vi "Example ADC PCF8591.vi"() -> ()   [LabVIEW 2014]
uses:
  vi.lib/Q-WaveSystems/QwaveSys Raspberry Pi for LabVIEW Home-Education/QwaveSys Raspberry Pi Library.lvlib
panel:
  in  "DAC":u8=77
  out "A3":i32
  out "A2":i32
  out "A1":i32
  out "A0":i32
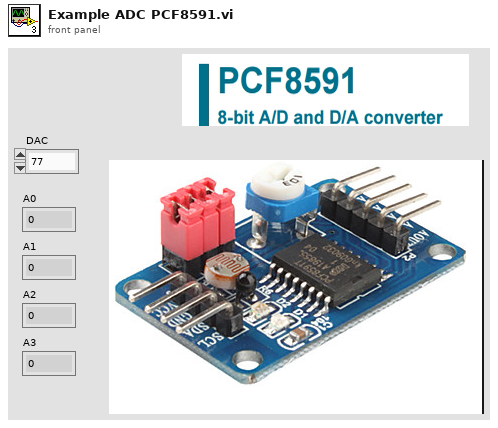
[diagram p1: front panel]
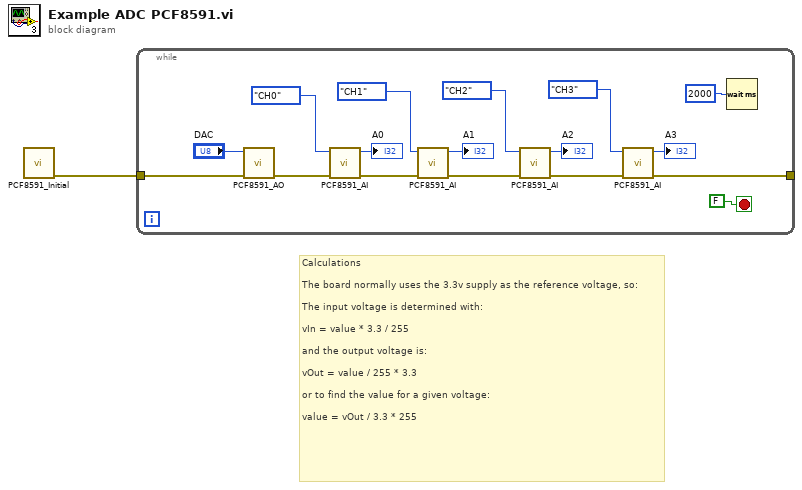
[diagram p0: block diagram]
diagram:
  # "Calculations\n\nThe board normally uses the 3.3v supply as the reference voltage, so:\n\nThe input voltage is determined with:\n\nvIn = value * 3.3 / 255\n\nand the output voltage is:\n\nvOut = value / 255 * 3.3\n\nor to find the value for a given voltage:\n\nvalue = vOut / 3.3 * 255"
  n1 = call "PCF8591_Initial.vi"() -> ("error out"=w1:errorcluster)  [unwired: 11 in]
  n2 = while {
    tunnel: w1 -> [w16]
    tunnel: [w7] -> _
    stop <- FALSE stop-if-true
    n3 = call "PCF8591_AO.vi"("error in (no error)"=w16, "DAC (0-255)"="DAC") -> ("error out"=w14:errorcluster)  [unwired: 9 in]
    n4 = call "PCF8591_AI.vi"("error in (no error)"=w14, "Channel"=enum16{"CH0", "CH1", "CH2", "CH3"}."CH0") -> ("error out"=w10:errorcluster, "Data"=→"A0":i32)  [unwired: 8 in]
    n5 = call "PCF8591_AI.vi"("error in (no error)"=w10, "Channel"=enum16{"CH0", "CH1", "CH2", "CH3"}."CH1") -> ("error out"=w9:errorcluster, "Data"=→"A1":i32)  [unwired: 8 in]
    n6 = call "PCF8591_AI.vi"("error in (no error)"=w9, "Channel"=enum16{"CH0", "CH1", "CH2", "CH3"}."CH2") -> ("error out"=w8:errorcluster, "Data"=→"A2":i32)  [unwired: 8 in]
    n7 = call "PCF8591_AI.vi"("error in (no error)"=w8, "Channel"=enum16{"CH0", "CH1", "CH2", "CH3"}."CH3") -> ("error out"=w7:errorcluster, "Data"=→"A3":i32)  [unwired: 8 in]
    n8 = Wait (ms)(milliseconds to wait=u32 2000) -> ()  [unwired: 1 out]
  }
